vi "add_JointCommand_roslv.vi"(8 "Mode":T1=1 items=["Position"=1, "Velocity"=2, "Effort"=3], 9 "names":string[](array[string]), 10 "command":dbl[](array[numeric]), 11 "msg in":string) -> (3 "msg out":string)   [LabVIEW 2014]
doc: "Flattens joint commands into a string"
uses:
  utils/JointMode.ctl
  std_msgs/subs/i32Scalar_roslv.vi
  std_msgs/subs/float64Array_roslv.vi
  std_msgs/subs/stringArray_roslv.vi
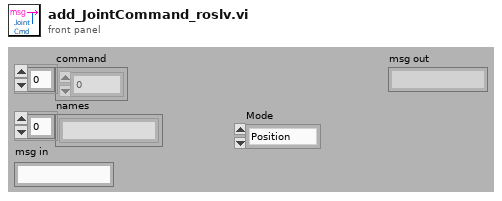
[diagram p1: front panel]
types:
  T1 = typedef "JointMode.ctl" = u8
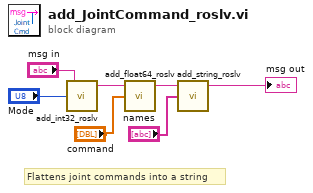
[diagram p0: block diagram]
diagram:
  # "Flattens joint commands into a string"
  n1 = call-poly "add_int32_roslv.vi"("Numeric"="Mode", "msg in"="msg in") -> ("msg out"=w7:string)  [unwired: 3 in]
  n2 = call-poly "add_float64_roslv.vi"("Array"="command", "msg in"=w7) -> ("msg out"=w6:string)  [unwired: 3 in]
  n3 = call-poly "add_string_roslv.vi"("Array"="names", "msg in"=w6) -> ("msg out"=→"msg out":string)  [unwired: 3 in]
